vi "Thev-Show Summary.vi"(0 "Data Folder":path, 5 "P0":refnum<vi>, 7 "Z0":refnum<vi>, 11 "error in (no error)":errorcluster) -> (15 "error out":errorcluster)   [LabVIEW 2015]
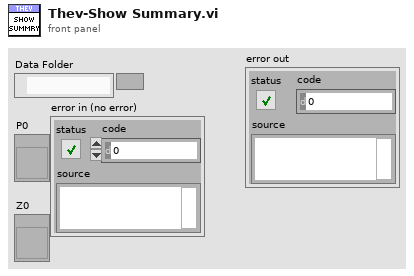
[diagram p1: front panel]
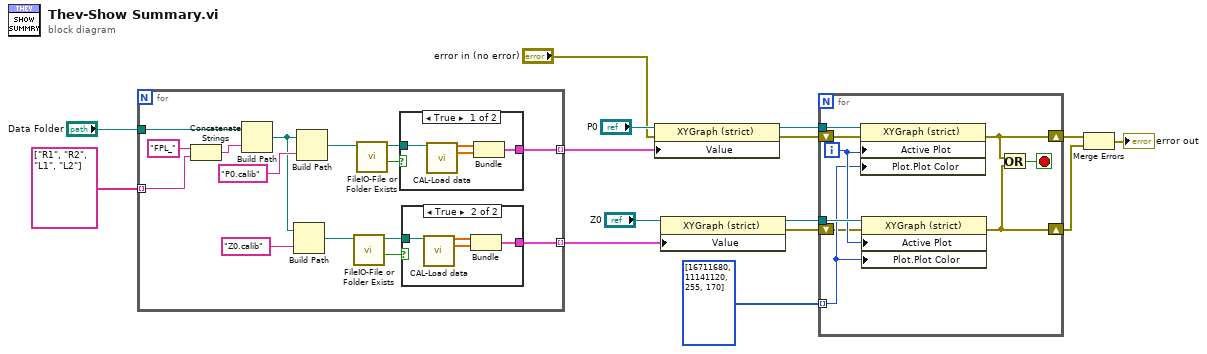
[diagram p0: block diagram]
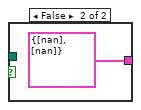
[diagram p2: hidden frame]
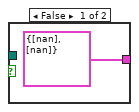
[diagram p3: hidden frame]
diagram:
  n1 = for {
    tunnel: "Data Folder" -> [w30]
    tunnel: string[] ["R1", "R2", "L1", "L2"] -> [w28] mode=indexing
    tunnel: [w17] -> w12 mode=indexing
    tunnel: [w16] -> w10 mode=indexing
    n2 = Concatenate Strings("FPL_", w28) -> (w27:string)
    n3 = Build Path(base path=w30, name or relative path=w27) -> (appended path=w19:path)
    n4 = Build Path(base path=w19, name or relative path="Z0.calib") -> (appended path=w20:path)
    n5 = Build Path(base path=w19, name or relative path="P0.calib") -> (appended path=w23:path)
    n6 = call "FileIO-File or Folder Exists.vi"("path"=w20) -> ("Exists?"=w21:bool, "dup path"=w22:path)  [unwired: 7 in, 2 out]
    n7 = call "FileIO-File or Folder Exists.vi"("path"=w23) -> ("Exists?"=w25:bool, "dup path"=w26:path)  [unwired: 7 in, 2 out]
    n8 = case shown="True" w25 {
      tunnel: w26 -> [w34 _]
      tunnel: [w31 cluster{dbl[], dbl[]} {[nan], [nan]} ("XY Data")] -> w17
      frame True {
        n9 = call "CAL-Load data.vi"("user path"=w34) -> ("Frequency (Hz)"=w32:dbl[], "Mag"=w33:dbl[])  [unwired: 7 in, 6 out]
        n10 = Bundle("Frequency (Hz)"=w32, "Mag"=w33) -> (w31:cluster{"Frequency (Hz)":dbl[], "Mag":dbl[]})  [unwired: 1 in]
      }
      frame False {
      }
    }
    n11 = case shown="True" w21 {
      tunnel: w22 -> [_ w40]
      tunnel: [cluster{dbl[], dbl[]} {[nan], [nan]} ("XY Data") w37] -> w16
      frame False {
      }
      frame True {
        n12 = call "CAL-Load data.vi"("user path"=w40) -> ("Frequency (Hz)"=w38:dbl[], "Mag"=w39:dbl[])  [unwired: 7 in, 6 out]
        n13 = Bundle("Frequency (Hz)"=w38, "Mag"=w39) -> (w37:cluster{"Frequency (Hz)":dbl[], "Mag":dbl[]})  [unwired: 1 in]
      }
    }
  }
  n14 = property class="XYGraph (strict)"(reference="P0", error in="error in (no error)", "Value"=w12) -> (reference out=w9:refnum<vi>, error out=w5:errorcluster)
  n15 = property class="XYGraph (strict)"(reference="Z0", "Value"=w10) -> (reference out=w8:refnum<vi>, error out=w4:errorcluster)  [unwired: 1 in]
  n16 = for {
    tunnel: w9 -> [w49]
    tunnel: w8 -> [w48]
    tunnel: u32[] [16711680, 11141120, 255, 170] -> [w46] mode=indexing
    shift-right: [w43] -> w3
    shift-left: w5 -> [w45]
    shift-right: [w42] -> w2
    shift-left: w4 -> [w44]
    i -> [w47]
    stop <- w41 stop-if-true
    n17 = property class="XYGraph (strict)"(reference=w49, error in=w45, "Active Plot"=w47, "Plot.Plot Color"=w46) -> (error out=w43:errorcluster)  [unwired: 1 out]
    n18 = property class="XYGraph (strict)"(reference=w48, error in=w44, "Active Plot"=w47, "Plot.Plot Color"=w46) -> (error out=w42:errorcluster)  [unwired: 1 out]
    n19 = Or(x=w43, y=w42) -> (x .or. y?=w41:bool)
  }
  n20 = Merge Errors(w3, w2) -> (→"error out":errorcluster)
